vi "PS_TapAverageCalc.vi"(2 "Period":dbl, 3 "DCI Array":u32[](array[numeric])=[86, 174, 265]) -> (1 "PS_TAP":dbl)   [LabVIEW 2018]
panel:
  out "DCI Array 2":u32[](array[numeric])=[86, 174, 265]
  out "DCI Array":u32[](array[numeric])=[86, 174, 265]
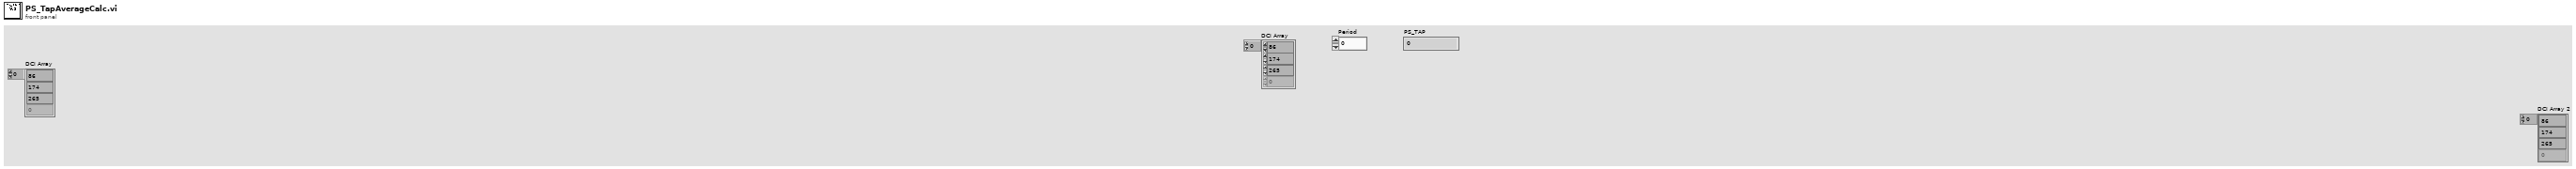
[diagram p1: front panel]
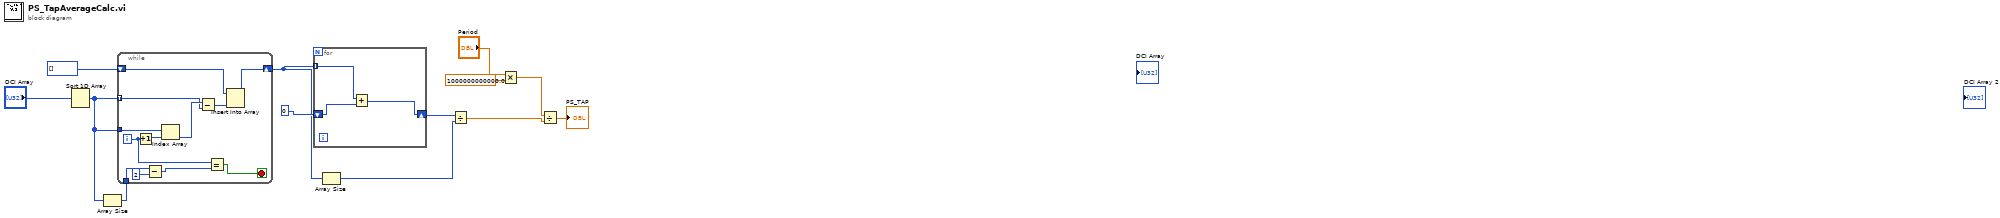
[diagram p0: block diagram]
diagram:
  n1 = Sort 1D Array(array="DCI Array") -> (sorted array=w2:u32[])
  n2 = Array Size(array=w2) -> (size(s)=w1:i32)
  n3 = while {
    tunnel: w2 -> [w22] mode=indexing
    tunnel: w2 -> [w24]
    shift-right: [w19] -> w9
    shift-left: u32[] [] -> [w20]
    tunnel: w1 -> [w16]
    i -> [w18]
    stop <- w17 stop-if-true
    n4 = Increment(x=w18) -> (x+1=w25:i32)
    n5 = Subtract(x=w16, y=2) -> (x-y=w14:i32)
    n6 = Index Array(array=w24, index=w25) -> (element=w23:u32)
    n7 = Subtract(x=w23, y=w22) -> (x-y=w21:u32)
    n8 = Equal?(x=w18, y=w14) -> (x = y?=w17:bool)
    n9 = Insert Into Array(array=w20, new element=w21) -> (w19:u32[])  [unwired: 1 in]
  }
  n10 = for {
    tunnel: w9 -> [w28] mode=indexing
    shift-right: [w26] -> w10
    shift-left: u32 0 -> [w27]
    n11 = Add(x=w28, y=w27) -> (x+y=w26:u32)
  }
  n12 = Array Size(array=w9) -> (size(s)=w8:i32)
  n13 = Divide(x=w10, y=w8) -> (x/y=w4:dbl)
  n14 = Multiply(x="Period", y=1000000000000.0) -> (x*y=w5:dbl)
  n15 = Divide(x=w5, y=w4) -> (x/y=→"PS_TAP":dbl)
